vi "TEST_DUMMY.vi"() -> ()   [LabVIEW 2019]
panel:
  in  "Dataflow In":errorcluster
  out "Dataflow Out":errorcluster
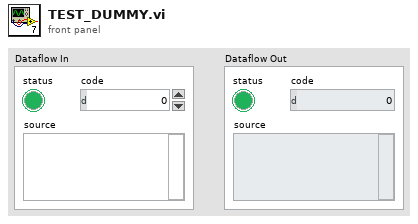
[diagram p1: front panel]
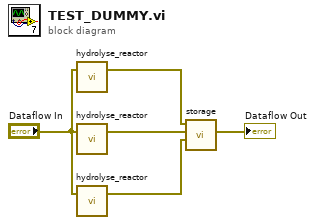
[diagram p0: block diagram]
diagram:
  n1 = call "hydrolyse_reactor.vi"("Dataflow In"="Dataflow In") -> ("Dataflow Out"=w4:errorcluster)  [unwired: 2 in]
  n2 = call "hydrolyse_reactor.vi"("Dataflow In"="Dataflow In") -> ("Dataflow Out"=w3:errorcluster)  [unwired: 2 in]
  n3 = call "hydrolyse_reactor.vi"("Dataflow In"="Dataflow In") -> ("Dataflow Out"=w2:errorcluster)  [unwired: 2 in]
  n4 = call "storage.vi"("Dataflow In #3"=w2, "Dataflow In #2"=w3, "Dataflow In #1"=w4) -> ("Dataflow Out"=→"Dataflow Out":errorcluster)  [unwired: 8 in]
